vi "Math-Diff.vi"(1 "X":dbl[](array[numeric])) -> (0 "diff(X)":dbl[](array[numeric]))   [LabVIEW 2020]
uses:
  <vilib>/Analysis/NI_AALPro.lvlib
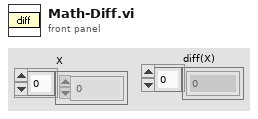
[diagram p1: front panel]
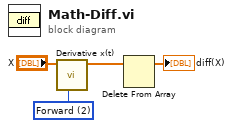
[diagram p0: block diagram]
diagram:
  w4 = u16 2 items=["2nd Order Central", "4th Order Central", "Forward", "Backward"] ("method")
  n1 = call <vilib>:"Derivative x(t).vi"("method"=w4, "X"="X") -> ("dX/dt"=w2:dbl[])  [unwired: 8 in, 1 out]
  n2 = Delete From Array(array=w2) -> (array with subset deleted=→"diff(X)":dbl[])  [unwired: 2 in, 1 out]
